vi "ConvertExperimentRunsToDisplayRuns.vi"(11 "Experiment Runs":T2[](array[typedef])) -> (3 "Display Runs":T1[](array[typedef]) {"Stop Current" format="%.3p"; "Start Current" format="%.3p"; "Stop Fluence" format="%.3e"; "Start Fluence" format="%.3e"; "Stop Dose" format="%.3e"; "Start Dose" format="%.3e"; "Stop Time" format="%<%H:%M:%S\n%m/%d/%Y>T"; "Start Time" format="%<%H:%M:%S\n%m/%d/%Y>T"})   [LabVIEW 2012]
uses:
  ExperimentRun.ctl
  ExperimentRunTiming.ctl
  ExperimentRunDose.ctl
  ExperimentRunFluence.ctl
  ExperimentRunTotalCharge.ctl
  DisplayRun.ctl
panel:
  # "Current"
  # "Stop"
  # "Start"
  # "Fluence"
  # "Stop"
  # "Start"
  # "Dose"
  # "Stop"
  # "Start"
  # "Timing"
  # "Stop"
  # "Start"
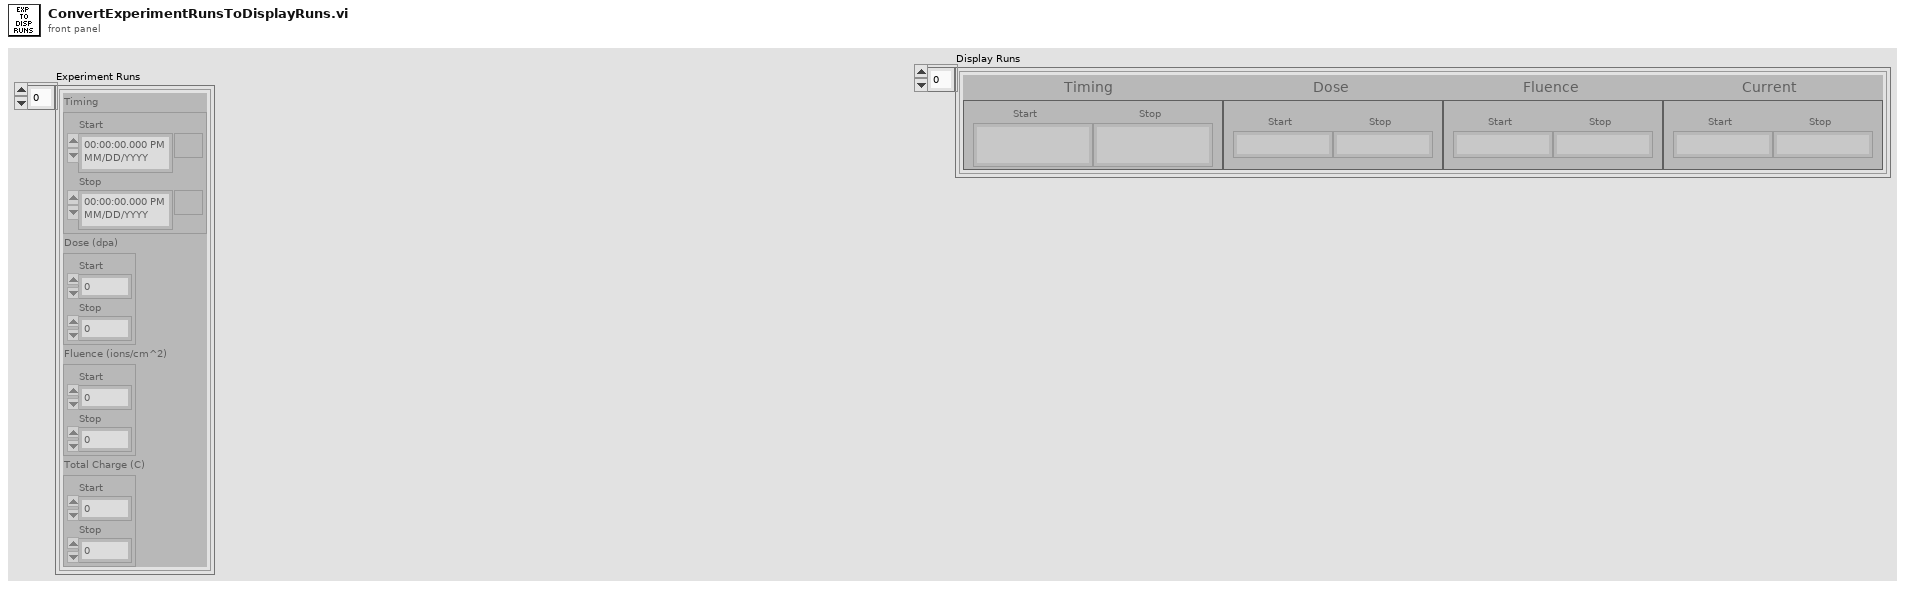
[diagram p1: front panel]
types:
  T1 = typedef "DisplayRun.ctl" = cluster{"Start Time":timestamp, "Stop Time":timestamp, "Start Dose":dbl, "Stop Dose":dbl, "Start Fluence":dbl, "Stop Fluence":dbl, "Start Current":dbl, "Stop Current":dbl}
  T2 = typedef "ExperimentRun.ctl" = cluster{"Timing":T3, "Dose (dpa)":T4, "Fluence (ions/cm^2)":T5, "Total Charge (C)":T6}
  T3 = typedef "ExperimentRunTiming.ctl" = cluster{"Start":timestamp, "Stop":timestamp}
  T4 = typedef "ExperimentRunDose.ctl" = cluster{"Start":dbl, "Stop":dbl}
  T5 = typedef "ExperimentRunFluence.ctl" = cluster{"Start":dbl, "Stop":dbl}
  T6 = typedef "ExperimentRunTotalCharge.ctl" = cluster{"Start":dbl, "Stop":dbl}
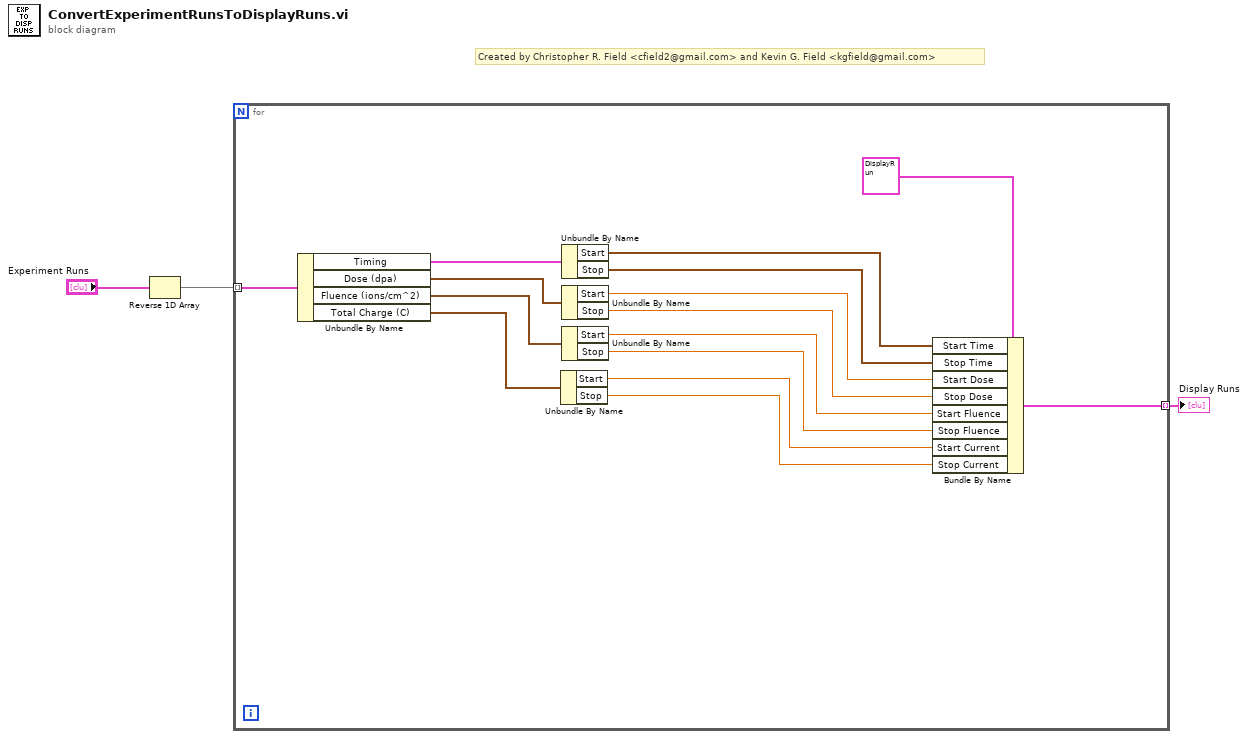
[diagram p0: block diagram]
diagram:
  # "Created by Christopher R. Field <cfield2@gmail.com> and Kevin G. Field <kgfield@gmail.com>"
  n1 = Reverse 1D Array(array="Experiment Runs") -> (reversed array=w1:T2[])
  n2 = for {
    tunnel: w1 -> [w18] mode=indexing
    tunnel: [w16] -> w3 mode=indexing
    n3 = Unbundle By Name(w18) -> ("Timing"=w15:T3, "Dose (dpa)"=w12:T4, "Fluence (ions/cm^2)"=w9:T5, "Total Charge (C)"=w6:T6)
    n4 = Unbundle By Name(w6) -> ("Start"=w5:dbl, "Stop"=w4:dbl)
    n5 = Unbundle By Name(w15) -> ("Start"=w14:timestamp, "Stop"=w13:timestamp)
    n6 = Unbundle By Name(w12) -> ("Start"=w11:dbl, "Stop"=w10:dbl)
    n7 = Unbundle By Name(w9) -> ("Start"=w8:dbl, "Stop"=w7:dbl)
    n8 = Bundle By Name(cluster=T1 {"Start Time"=timestamp(0 s since 1904-01-01), "Stop Time"=timestamp(0 s since 1904-01-01), "Start Dose"=0.0, "Stop Dose"=0.0, "Start Fluence"=0.0, "Stop Fluence"=0.0, "Start Current"=0.0, "Stop Current"=0.0} ("Experiment Run"), "Start Time"=w14, "Stop Time"=w13, "Start Dose"=w11, "Stop Dose"=w10, "Start Fluence"=w8, "Stop Fluence"=w7, "Start Current"=w5, "Stop Current"=w4) -> (w16:T1)
  }
  "Display Runs" <- w3
